vi "Get Int.vi"(8 "error in (no error)":errorcluster, 11 "IIntByRef in":refnum<class "IIntByRef (Unnamed SEQ).lvclass">) -> (0 "error out":errorcluster, 2 "Int":i32, 3 "IIntByRef out":refnum<class "IIntByRef (Unnamed SEQ).lvclass">)   [LabVIEW 2009, in "IIntByRef (Unnamed SEQ).lvclass"]
uses:
  IIntByRef (Unnamed SEQ).lvclass
  Numeric Test Object.lvclass
  Source/IUnknown Class/IUnknown.lvclass
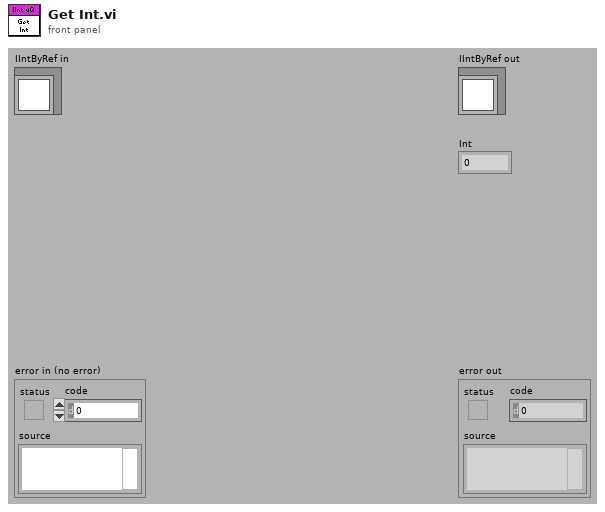
[diagram p1: front panel]
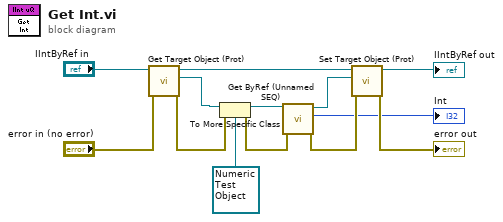
[diagram p0: block diagram]
diagram:
  n1 = call "Get Target Object (Prot).vi"("error in (no error)"="error in (no error)", "IUnknown in"="IIntByRef in") -> ("error out"=w12:errorcluster, "Target Object"=w13:refnum<class "Interfaceable.lvclass">, "IUnknown out"=w7:refnum<class "IIntByRef (Unnamed SEQ).lvclass">)  [unwired: 7 in]
  n2 = To More Specific Class(target class=refnum<class "Numeric Test Object.lvclass"> refnum ("Numeric"), reference=w13, error in=w12) -> (specific class reference=w10:refnum<class "Numeric Test Object.lvclass">, error out=w9:errorcluster)
  n3 = call-dynamic "Get ByRef (Unnamed SEQ).vi"("error in (no error)"=w9, "Numeric in"=w10) -> ("error out"=w6:errorcluster, "Int"=→"Int":i32, "Numeric out"=w8:refnum<class "Numeric Test Object.lvclass">)  [unwired: 7 in]
  n4 = call "Set Target Object (Prot).vi"("error in (no error)"=w6, "Target Object"=w8, "IUnknown in"=w7) -> ("error out"=→"error out":errorcluster, "IUnknown out"=→"IIntByRef out":refnum<class "IIntByRef (Unnamed SEQ).lvclass">)  [unwired: 7 in]
